vi "Pre Launch Init.vi"(11 "Nested in":refnum<class "UI Actor.lvclass">) -> (0 "error out":errorcluster, 3 "Nested out":refnum<class "UI Actor.lvclass">)   [LabVIEW 2020, in "UI Actor.lvlib" / "UI Actor.lvclass"]
doc: "(<B>Filename</B>: Actor Framework.lvlib:Actor.lvclass:Pre Launch Init.vi)\n\nDefines behavior that occurs after the Launch Nested Actor method is invoked but before the actor's Actor Core method begins running.\n\nBy default, this method does nothing. A descendant class may override it to define behavior."
uses:
  UI Actor.lvclass
  C:/Program Files (x86)/National Instruments/LabVIEW 2020/vi.lib/ActorFramework/Actor/Actor.lvclass
  UI Actor.lvclass/UI Actor.ctl
  <vilib>/ActorFramework/Actor/Actor.lvclass/Actor.ctl
  <vilib>/ActorFramework/Message Enqueuer/Message Enqueuer.lvclass/Message Enqueuer.ctl
  <vilib>/ActorFramework/Message Enqueuer/Init from Existing Queue.vi
  <vilib>/ActorFramework/Message Enqueuer/Enqueue.vi
  UI Actor Messages/Init Msg/Init Msg.lvclass
  C:/Program Files (x86)/National Instruments/LabVIEW 2020/vi.lib/ActorFramework/Message/Message.lvclass
  <vilib>/ActorFramework/Message Priority Queue/Priority Enqueue.vi
  <vilib>/ActorFramework/Message Enqueuer/Message Enqueuer.lvclass
  <vilib>/ActorFramework/Actor/Actor.lvclass
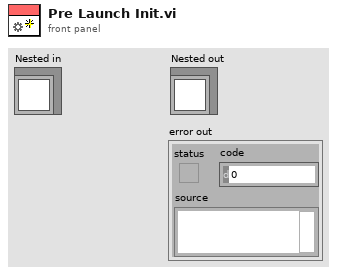
[diagram p1: front panel]
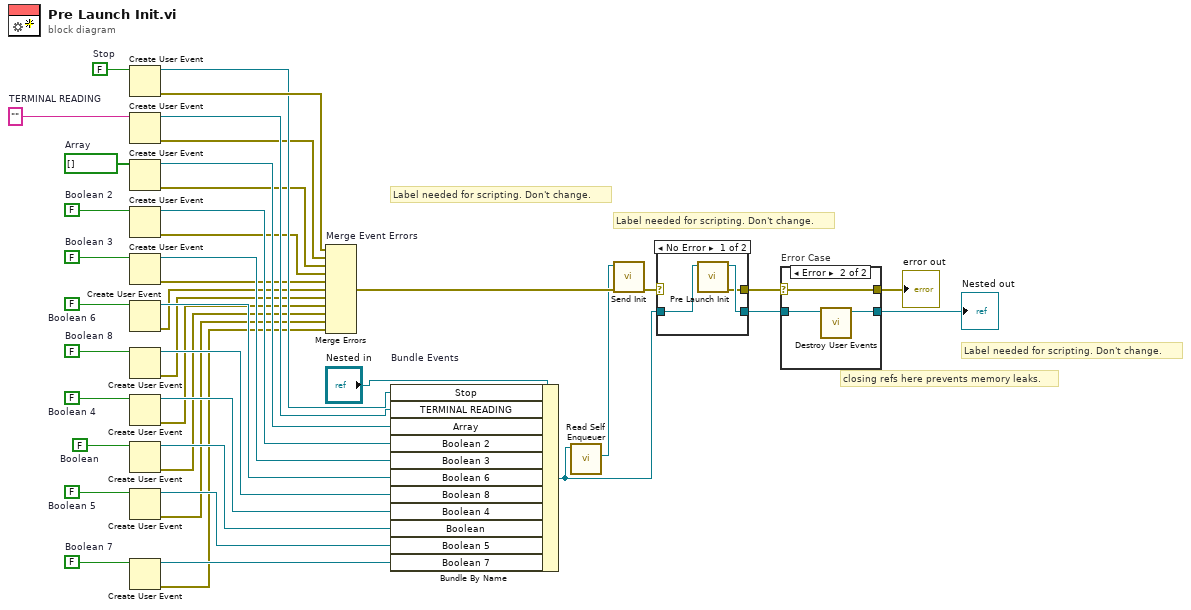
[diagram p0: block diagram]
diagram:
  w3 = FALSE  # Boolean 7
  w6 = FALSE  # Boolean 5
  w9 = FALSE  # Boolean
  w12 = FALSE  # Boolean 4
  w15 = FALSE  # Boolean 8
  w18 = FALSE  # Boolean 6
  w21 = FALSE  # Boolean 3
  w24 = FALSE  # Boolean 2
  w27 = bool[] []  # Array
  w30 = ""  # TERMINAL READING
  w41 = FALSE  # Stop
  # "Label needed for scripting. Don't change."
  # "Label needed for scripting. Don't change."
  # "Label needed for scripting. Don't change."
  # "closing refs here prevents memory leaks."
  n1 = Create User Event(user event datatype=w41) -> (user event=w38:refnum<user-event>, error out=w40:errorcluster)  [unwired: 1 in]
  n2 = Create User Event(user event datatype=w30) -> (user event=w29:refnum<user-event>, error out=w28:errorcluster)  [unwired: 1 in]
  n3 = Create User Event(user event datatype=w27) -> (user event=w26:refnum<user-event>, error out=w25:errorcluster)  [unwired: 1 in]
  n4 = Create User Event(user event datatype=w24) -> (user event=w23:refnum<user-event>, error out=w22:errorcluster)  [unwired: 1 in]
  n5 = Create User Event(user event datatype=w21) -> (user event=w20:refnum<user-event>, error out=w19:errorcluster)  [unwired: 1 in]
  n6 = Create User Event(user event datatype=w18) -> (user event=w17:refnum<user-event>, error out=w16:errorcluster)  [unwired: 1 in]
  n7 = Create User Event(user event datatype=w15) -> (user event=w14:refnum<user-event>, error out=w13:errorcluster)  [unwired: 1 in]
  n8 = Create User Event(user event datatype=w12) -> (user event=w11:refnum<user-event>, error out=w10:errorcluster)  [unwired: 1 in]
  n9 = Create User Event(user event datatype=w9) -> (user event=w8:refnum<user-event>, error out=w7:errorcluster)  [unwired: 1 in]
  n10 = Create User Event(user event datatype=w6) -> (user event=w5:refnum<user-event>, error out=w4:errorcluster)  [unwired: 1 in]
  n11 = Create User Event(user event datatype=w3) -> (user event=w2:refnum<user-event>, error out=w1:errorcluster)  [unwired: 1 in]
  n12 = Merge Errors "Merge Event Errors"(w40, w28, w25, w22, w19, w16, w13, w10, w7, w4, w1) -> (w32:errorcluster)
  n13 = Bundle By Name "Bundle Events"(cluster="Nested in", "Stop"=w38, "TERMINAL READING"=w29, "Array"=w26, "Boolean 2"=w23, "Boolean 3"=w20, "Boolean 6"=w17, "Boolean 8"=w14, "Boolean 4"=w11, "Boolean"=w8, "Boolean 5"=w5, "Boolean 7"=w2) -> (w34:refnum<class "UI Actor.lvclass">)
  n14 = call <vilib>:"Read Self Enqueuer.vi"("Actor"=w34) -> ("Self Enqueuer"=w31:refnum<class "Message Enqueuer.lvclass">)  [unwired: 10 in]
  n15 = call "Send Init.vi"("error in (no error)"=w32, "Message Enqueuer"=w31) -> ("error out"=w33:errorcluster)  [unwired: 8 in, 1 out]
  n16 = case shown="No Error" w33 {
    selector: w33 -> [_ w47]
    tunnel: [w45 w46] -> w36
    tunnel: w34 -> [w44 w46]
    tunnel: [w43 w47] -> w35
    frame No Error {
      n17 = call-parent "Pre Launch Init.vi"("Actor in"=w44) -> ("error out"=w43:errorcluster, "Actor out"=w45:refnum<class "UI Actor.lvclass">)  [unwired: 9 in]
    }
    frame Error {
    }
  }
  n18 = case "Error Case" shown="Error" w35 {
    selector: w35 -> [w48 w52]
    tunnel: w36 -> [w49 w51]
    tunnel: [w49 w50] -> w39
    tunnel: [w48 w52] -> w37
    frame No Error {
    }
    frame Error {
      n19 = call "Destroy User Events.vi"("UI Template in"=w51) -> ("UI Template out"=w50:refnum<class "UI Actor.lvclass">)  [unwired: 10 in]
    }
  }
  "error out" <- w37
  "Nested out" <- w39
